vi "Get_Live_Image_Sub.vi"(3 "error in":errorcluster, 4 "index":i32, 5 "Session Array":T2[](array[typedef])) -> (0 "error out":errorcluster, 2 "Image":T1(plugin-control))   [LabVIEW 2022 SP3]
uses:
  <vilib>/vision/driver/IMAQdx.llb/IMAQdx Buffer Number Mode.ctl
  Picture Display Global.vi
  Camera Server/Globals/CamServer global.vi
  <vilib>/userDefined/High Color/IMAQdx.ctl
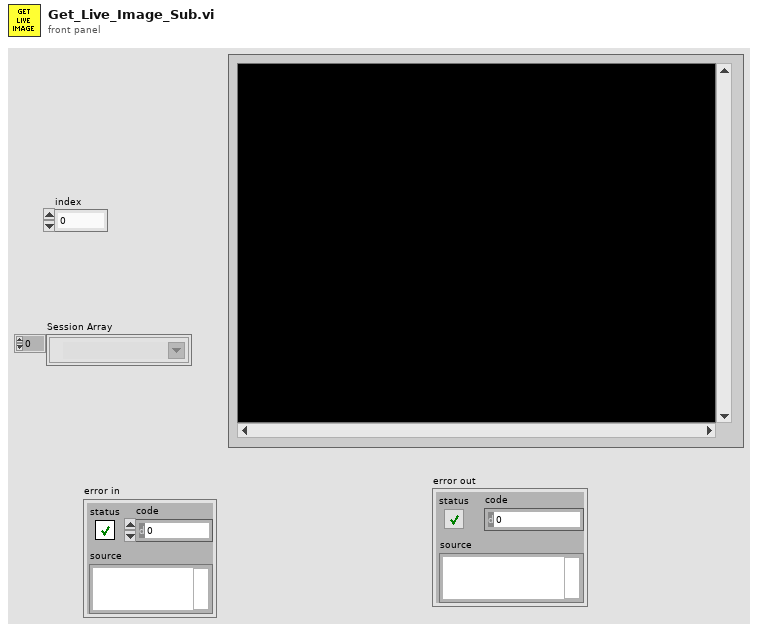
[diagram p1: front panel]
types:
  T1 = typedef "IMAQ Image.ctl" = refnum<image>
  T2 = typedef "IMAQdx.ctl" = refnum<k21>
  T3 = typedef "Camera enum.ctl" = string
  T4 = typedef "NI_Vision_Acquisition_Software.lvlib/IMAQdx Buffer Number Mode.ctl" = enum32{"Next", "Last", "Buffer Number", "Every", "Last New"}
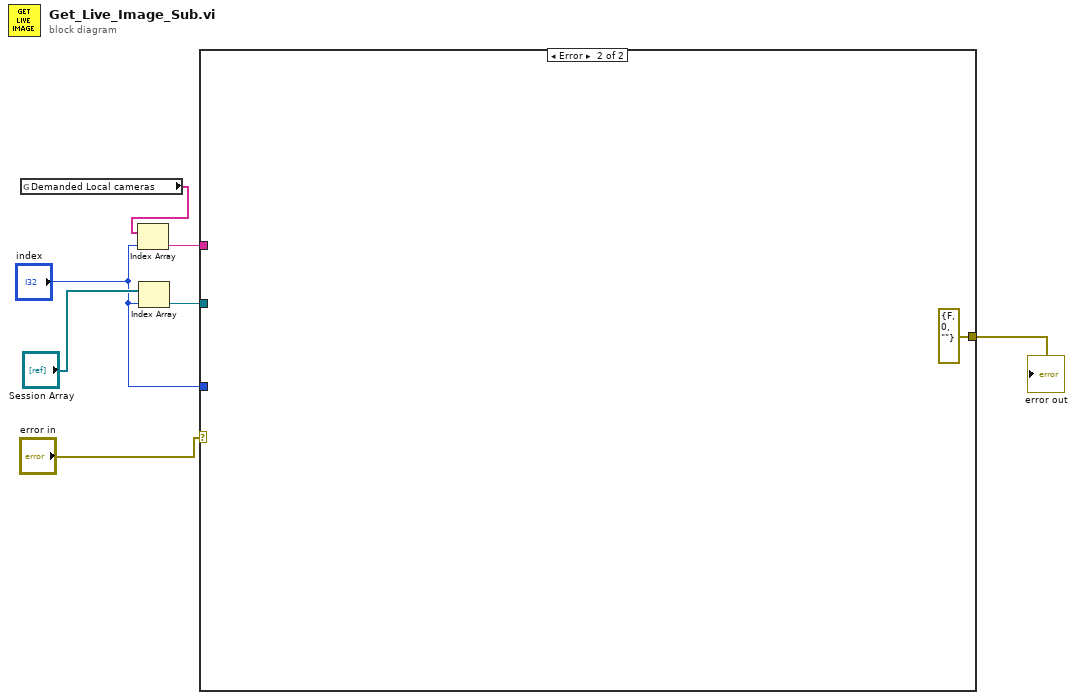
[diagram p0: block diagram]
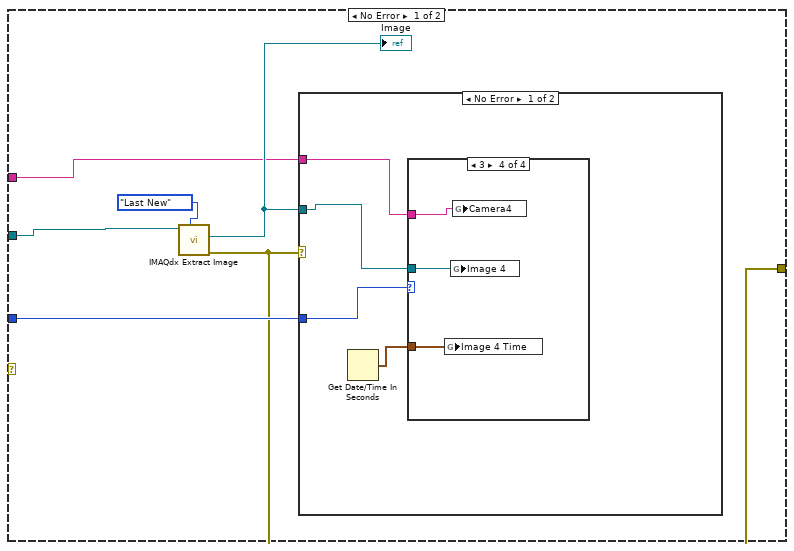
[diagram p2: hidden frame]
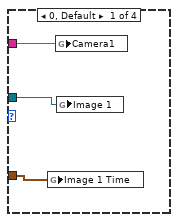
[diagram p3: hidden frame]
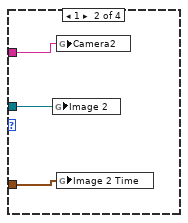
[diagram p4: hidden frame]
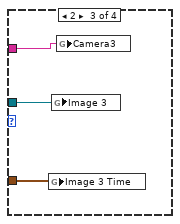
[diagram p5: hidden frame]
diagram:
  n1 = global read "CamServer global.vi" "Demanded Local cameras"() -> (w2:T3[])
  n2 = Index Array(array=w2, index="index") -> (element=w1:T3)
  n3 = Index Array(array="Session Array", index="index") -> (element=w7:T2)
  n4 = case shown="Error" "error in" {
    tunnel: w7 -> [w13 _]
    tunnel: [w9 errorcluster {"status"=FALSE, "code"=0, "source"=""} ("error out")] -> w5
    tunnel: "index" -> [w11 _]
    tunnel: w1 -> [w8 _]
    frame No Error {
      n5 = call <vilib>:"IMAQdx Extract Image.vi"("Buffer Number Mode (Next)"=IMAQdx_Buffer_Number_Mode."Last New" ("Buffer Number Mode"), "Session In"=w13) -> ("error out"=w9:errorcluster, "Image Out"=w10:T1)  [unwired: 6 in, 2 out]
      "Image" <- w10
      n6 = case shown="No Error" w9 {
        tunnel: w11 -> [w17 _]
        tunnel: w10 -> [w16 _]
        tunnel: w8 -> [w14 _]
        frame No Error {
          n7 = Get Date/Time In Seconds() -> (seconds since 1Jan1904=w15:timestamp)
          n8 = case shown="3" w17 {
            tunnel: w16 -> [w19 w22 w25 w29]
            tunnel: w15 -> [w20 w23 w26 w28]
            tunnel: w14 -> [w18 w21 w24 w27]
            frame 0, Default {
              n9 = global write "Picture Display Global.vi" "Image 1 Time"(w20) -> ()
              n10 = global write "Picture Display Global.vi" "Camera1"(w18) -> ()
              n11 = global write "Picture Display Global.vi" "Image 1"(w19) -> ()
            }
            frame 1 {
              n12 = global write "Picture Display Global.vi" "Image 2"(w22) -> ()
              n13 = global write "Picture Display Global.vi" "Camera2"(w21) -> ()
              n14 = global write "Picture Display Global.vi" "Image 2 Time"(w23) -> ()
            }
            frame 2 {
              n15 = global write "Picture Display Global.vi" "Image 3 Time"(w26) -> ()
              n16 = global write "Picture Display Global.vi" "Image 3"(w25) -> ()
              n17 = global write "Picture Display Global.vi" "Camera3"(w24) -> ()
            }
            frame 3 {
              n18 = global write "Picture Display Global.vi" "Image 4 Time"(w28) -> ()
              n19 = global write "Picture Display Global.vi" "Image 4"(w29) -> ()
              n20 = global write "Picture Display Global.vi" "Camera4"(w27) -> ()
            }
          }
        }
        frame Error {
        }
      }
    }
    frame Error {
    }
  }
  "error out" <- w5
